vi "queueAcq.vi"(7 "New trial":bool, 8 "error in (no error)":errorcluster, 9 "stimulus":string, 10 "trial":dbl, 11 "Acquisition in":refnum<class "Acquisition.lvclass">) -> (0 "error out":errorcluster, 2 "current time":timestamp, 3 "Acquisition out":refnum<class "Acquisition.lvclass">)   [LabVIEW 2014, in "Acquisition.lvclass"]
uses:
  Acquisition.lvclass
  Acquisition.lvclass/Acquisition.ctl
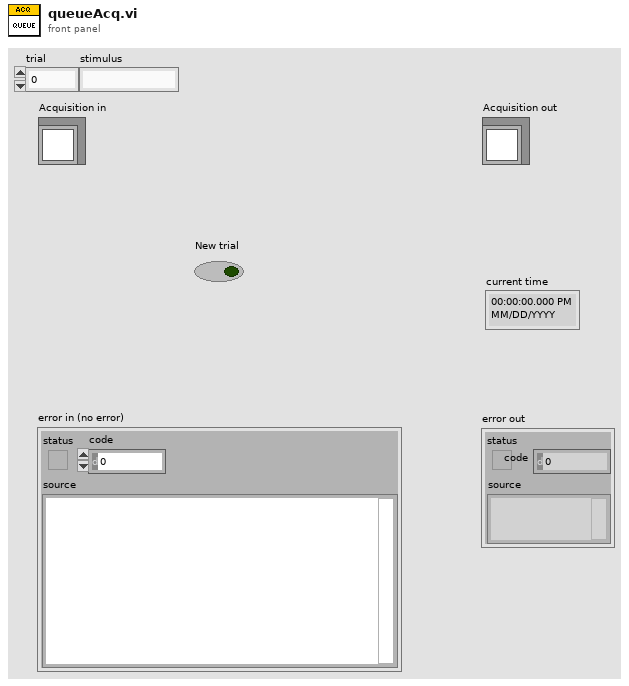
[diagram p1: front panel]
types:
  T1 = cluster{"timestamp":dbl, "stimulus":string, "trial":dbl}
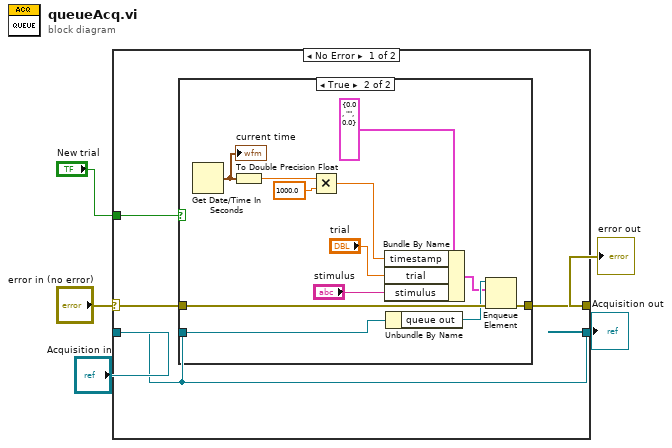
[diagram p0: block diagram]
diagram:
  n1 = case shown="No Error" "error in (no error)" {
    selector: "error in (no error)" -> [w9 w24]
    tunnel: [w8 w24] -> w4
    tunnel: [w7 w23] -> w2
    tunnel: "Acquisition in" -> [w7 w23]
    tunnel: "New trial" -> [w6 _]
    frame No Error {
      n2 = case shown="True" w6 {
        tunnel: w9 -> [w10 w19]
        tunnel: [w10 w18] -> w8
        tunnel: w7 -> [_ w16]
        frame False {
        }
        frame True {
          n3 = Get Date/Time In Seconds() -> (seconds since 1Jan1904=w20:timestamp)
          "current time" <- w20
          n4 = To Double Precision Float(number=w20) -> (double precision float=w21:dbl)
          n5 = Multiply(x=w21, y=1000.0) -> (x*y=w17:dbl)
          n6 = Bundle By Name(cluster=T1 {"timestamp"=0.0, "stimulus"="", "trial"=0.0} ("element"), "timestamp"=w17, "trial"="trial", "stimulus"="stimulus") -> (w11:T1)
          n7 = Unbundle By Name(w16) -> ("queue out"=w15:refnum<queue>)
          n8 = Enqueue Element(queue=w15, element=w11, error in (no error)=w19) -> (error out=w18:errorcluster)  [unwired: 1 in, 2 out]
        }
      }
    }
    frame Error {
    }
  }
  "error out" <- w4
  "Acquisition out" <- w2
